vi "PCO_WhiteBalanceToDisplayStruct.vi"(0 "ph":u64, 1 "gb12":u16[][](array[numeric])=array1x4097[4097 elements], 2 "y_min":i32, 3 "y_max":i32, 5 "mode":i32, 7 "width":i32, 9 "height":i32, 11 "error in (no error)":errorcluster {"code" format="%x"}, 12 "x_min":i32, 13 "x_max":i32) -> (4 "ph out":u64, 6 "ErrorMessage":i32 format="%x", 8 "strDisplay":T1, 15 "error out":errorcluster {"code" format="%x"})   [LabVIEW 2019, in "Convert.lvlib"]
doc: "int PCOCONVERT_API PCO_WhiteBalanceToDisplayStruct(HANDLE ph, PCO_Display* strDisplay, int mode, int width, int height,\n word *gb12, int x_min, int y_min, int x_max, int y_max);"
uses:
  Convert.lvlib
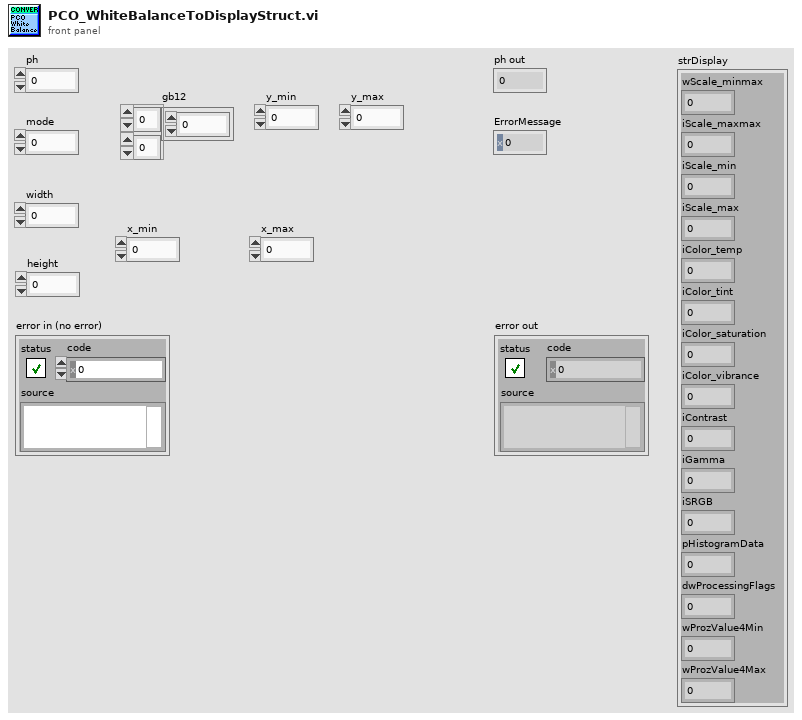
[diagram p1: front panel]
types:
  T1 = cluster{"wScale_minmax":u16, "iScale_maxmax":i32, "iScale_min":i32, "iScale_max":i32, "iColor_temp":i32, "iColor_tint":i32, "iColor_saturation":i32, "iColor_vibrance":i32, "iContrast":i32, "iGamma":i32, "iSRGB":i32, "pHistogramData":u64, "dwProcessingFlags":u32, "wProzValue4Min":u16, "wProzValue4Max":u16}
  T2 = cluster{"wSize":u16, "wScale_minmax":u16, "iScale_maxmax":i32, "iScale_min":i32, "iScale_max":i32, "iColor_temp":i32, "iColor_tint":i32, "iColor_saturation":i32, "iColor_vibrance":i32, "iContrast":i32, "iGamma":i32, "iSRGB":i32, "pHistogramData":u64, "dwDialogOpenFlags":u32, "dwProcessingFlags":u32, "wProzValue4Min":u16, "wProzValue4Max":u16, "dwzzDummy1":cluster{u32, u32, u32, u32, u32, u32, u32, u32, u32, u32, u32, u32, u32, u32, u32, u32, u32, u32, u32, u32, u32, u32, u32, u32, u32, u32, u32, u32, u32, u32, u32, u32, u32, u32, u32, u32, u32, u32, u32, u32, u32, u32, u32, u32, u32, u32, u32, u32, u32, u32}}
  T3 = cluster{"wSize":u16, "wScale_minmax":u16, "iScale_maxmax":i32, "iScale_min":i32, "iScale_max":i32, "iColor_temp":i32, "iColor_tint":i32, "iColor_saturation":i32, "iColor_vibrance":i32, "iContrast":i32, "iGamma":i32, "iSRGB":i32, "pHistogramData":u32, "dwDialogOpenFlags":u32, "dwProcessingFlags":u32, "wProzValue4Min":u16, "wProzValue4Max":u16, "dwzzDummy1":cluster{u32, u32, u32, u32, u32, u32, u32, u32, u32, u32, u32, u32, u32, u32, u32, u32, u32, u32, u32, u32, u32, u32, u32, u32, u32, u32, u32, u32, u32, u32, u32, u32, u32, u32, u32, u32, u32, u32, u32, u32, u32, u32, u32, u32, u32, u32, u32, u32, u32}}
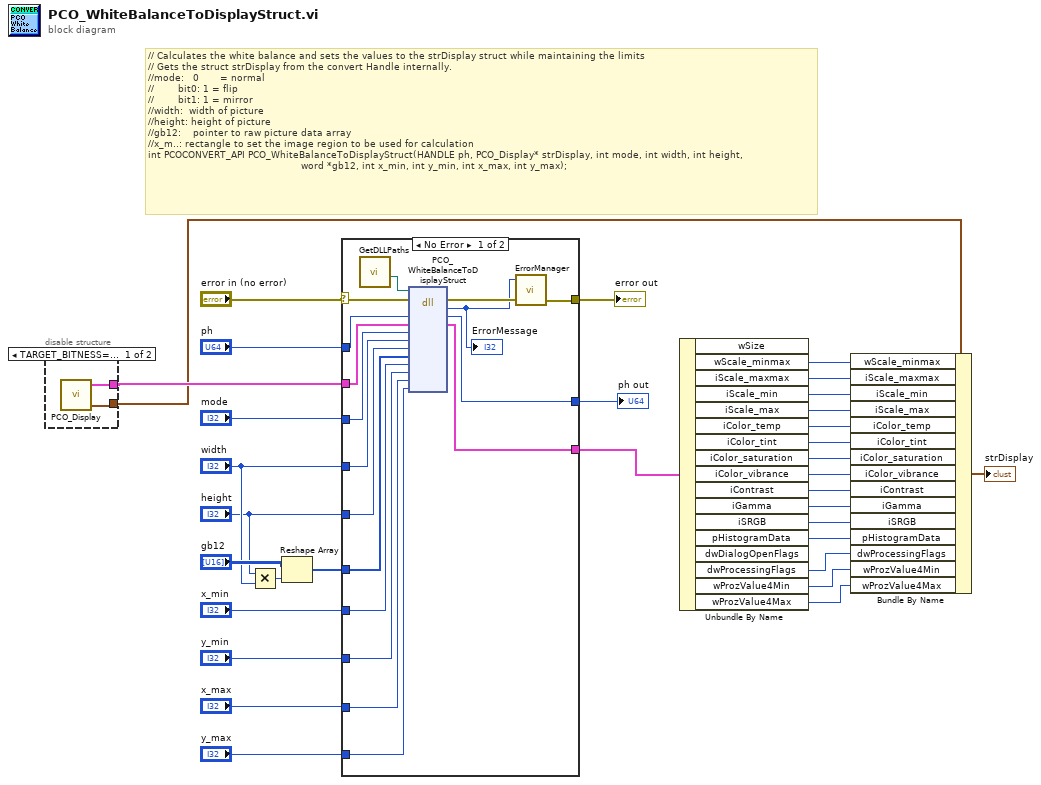
[diagram p0: block diagram]
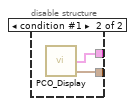
[diagram p2: hidden frame]
diagram:
  # "// Calculates the white balance and sets the values to the strDisplay struct while maintaining the limits\n// Gets the struct strDisplay from the convert Handle internally.\n//mode:   0       = normal\n//        bit0: 1 = flip\n//        bit1: 1 = mirror  \n//width:  width of picture\n//height: height of picture\n//gb12:    pointer to raw picture data array\n//x_m..: rectangle to set the image region to be used for calculation\nint PCOCONVERT_API PCO_WhiteBalanceToDisplayStruct(HANDLE ph, PCO_Display* strDisplay, int mode, int width, int height,\n                                                   word *gb12, int x_min, int y_min, int x_max, int y_max);"
  n1 = disable-structure "Diagram Disable Structure" shown="TARGET_BITNESS==64, Default" {
    disable-tunnel: [w35 w37] -> w22
    disable-tunnel: [w34 w36] -> w24
    frame condition #0 (active) {
      n2 = call "PCO_Display.vi"() -> ("PCO_DisplayRaw_x64"=w34:T2, "PCO_Display"=w35:T1)  [unwired: 4 in, 3 out]
    }
    frame condition #1 {
      n3 = call "PCO_Display.vi"() -> ("PCO_DisplayRaw_win32"=w36:T3, "PCO_Display"=w37:T1)  [unwired: 4 in, 3 out]
    }
  }
  n4 = Multiply(x="height", y="width") -> (x*y=w8:i32)
  n5 = Reshape Array("gb12", w8) -> (w5:u16[])
  n6 = case shown="No Error" "error in (no error)" {
    selector: "error in (no error)" -> [w43 w55]
    tunnel: "ph" -> [w54 w56]
    tunnel: [w53 w56] -> w32
    tunnel: [w52 w57] -> w23
    tunnel: "mode" -> [w51 _]
    tunnel: "width" -> [w50 _]
    tunnel: "height" -> [w49 _]
    tunnel: w5 -> [w48 _]
    tunnel: "x_min" -> [w47 _]
    tunnel: "y_min" -> [w46 _]
    tunnel: "x_max" -> [w45 _]
    tunnel: "y_max" -> [w44 _]
    tunnel: [w41 w55] -> w26
    tunnel: w24 -> [w39 w57]
    frame No Error {
      n7 = call "GetDLLPaths.vi"() -> ("PCO_Conv_Path"=w38:path)  [unwired: 8 in, 3 out]
      n8 = dll-call lib="?" fn="PCO_WhiteBalanceToDisplayStruct"(path in=w38, error in=w43, "ph"=w54, "strDisplay"=w39, "mode"=w51, "width"=w50, "height"=w49, "gb12"=w48, "x_min"=w47, "y_min"=w46, "x_max"=w45, "y_max"=w44) -> (error out=w42:errorcluster, "return type"=w40:i32, "ph"=w53:u64, "strDisplay"=w52:T2)  [unwired: 9 in, 1 out]
      "ErrorMessage" <- w40
      n9 = call "ErrorManager.vi"("error in (no error)"=w42, "error code"=w40) -> ("error out"=w41:errorcluster)  [unwired: 2 in, 1 out]
    }
    frame Error {
    }
  }
  "ph out" <- w32
  "error out" <- w26
  n10 = Unbundle By Name(w23) -> ("wScale_minmax"=w21:u16, "iScale_maxmax"=w20:i32, "iScale_min"=w19:i32, "iScale_max"=w18:i32, "iColor_temp"=w17:i32, "iColor_tint"=w16:i32, "iColor_saturation"=w15:i32, "iColor_vibrance"=w14:i32, "iContrast"=w13:i32, "iGamma"=w12:i32, "iSRGB"=w11:i32, "pHistogramData"=w10:u64, "dwProcessingFlags"=w4:u32, "wProzValue4Min"=w3:u16, "wProzValue4Max"=w2:u16)  [unwired: 2 out]
  n11 = Bundle By Name(cluster=w22, "wScale_minmax"=w21, "iScale_maxmax"=w20, "iScale_min"=w19, "iScale_max"=w18, "iColor_temp"=w17, "iColor_tint"=w16, "iColor_saturation"=w15, "iColor_vibrance"=w14, "iContrast"=w13, "iGamma"=w12, "iSRGB"=w11, "pHistogramData"=w10, "dwProcessingFlags"=w4, "wProzValue4Min"=w3, "wProzValue4Max"=w2) -> (→"strDisplay":T1)
